vi "InitializeSystemHealthTags.vi"(8 "error in (no error)":errorcluster) -> (0 "error out":errorcluster, 3 "health tags":T1[](array[typedef]))   [LabVIEW 2017, in "DeviceHealth.lvlib"]
uses:
  <vilib>/addons/InsightCM/Devices/Shared/Common/DeviceHealth/DeviceHealth.lvlib
  <vilib>/addons/InsightCM/Devices/Shared/Common/DeviceHealth/controls/deviceHealthTag.ctl
  <vilib>/addons/InsightCM/Devices/Shared/Common/DeviceHealth/controls/SystemHealthTagEnum.ctl
  <vilib>/addons/InsightCM/MessageBus/Base/controls/Tag.ctl
  <vilib>/addons/InsightCM/MessageBus/Base/controls/KeyValuePair.ctl
  <vilib>/addons/InsightCM/Utilities/GlobalConfiguration/GlobalConfiguration.lvlib
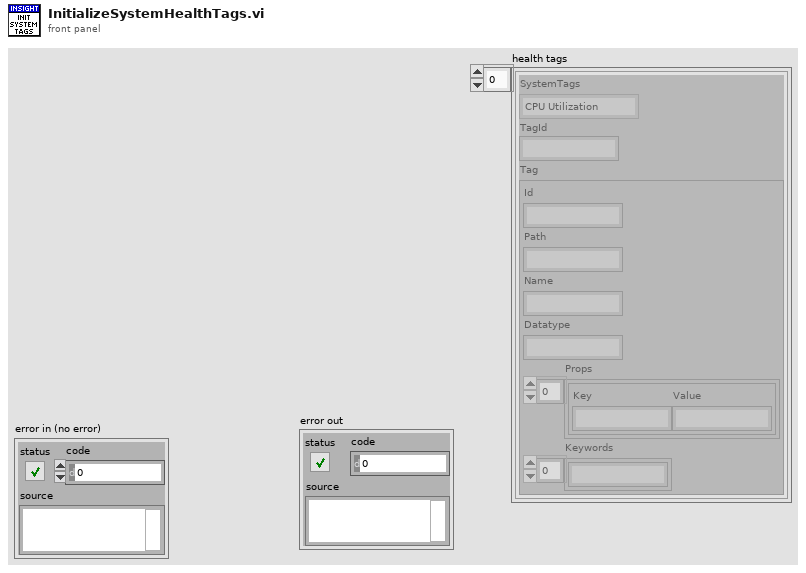
[diagram p1: front panel]
types:
  T1 = typedef "DeviceHealth.lvlib/deviceHealthTag.ctl" = cluster{"SystemTags":T2, "TagId":string, "Tag":T3}
  T2 = typedef "DeviceHealth.lvlib/SystemHealthTagEnum.ctl" = enum16{"CPU Utilization", "Memory Utilization", "Disk Utilization", "Total Physical Memory", "Primary Disk Free", "Chassis Temperature", "LowRateCount"}
  T3 = typedef "Tag.ctl" = cluster{"Id":string, "Path":string, "Name":string, "Datatype":string, "Props":T4[], "Keywords":string[]}
  T4 = typedef "KeyValuePair.ctl" = cluster{"Key":string, "Value":string}
  T5 = typedef "R2_Device.ctl" = cluster{"Id":string, "Name":string, "DeviceType":string, "HardwareName":string, "IpAddress":string, "HardwareInfo":T4[], "ApplicationType":string, "ApplicationVersion":string, "EquipmentIds":string[], "ConfigurationVersion":string, "State":T6, "Properties":T4[], "DataGroups":T7[], "BurstModeTrigger":T11}
  T6 = typedef "DeviceState.ctl" = cluster{"Disabled":bool}
  T7 = typedef "R2_DataGroup.ctl" = cluster{"Name":string, "OperatingStates":T8[], "Properties":T4[], "EquipmentIds":string[], "AssetNodeId":string}
  T8 = typedef "OperatingState.ctl" = cluster{"Name":string, "Properties":T4[], "Triggers":T9[]}
  T9 = typedef "Trigger.ctl" = cluster{"Type":string, "Expression":string, "Conditions":T10[]}
  T10 = typedef "Condition.ctl" = cluster{"Source":string, "Type":string, "Operator":string, "CompareTo":string, "DwellSeconds":dbl}
  T11 = typedef "BurstModeTrigger.ctl" = cluster{"Trigger":T9, "SampleRate":string, "AcquisitionLength":string}
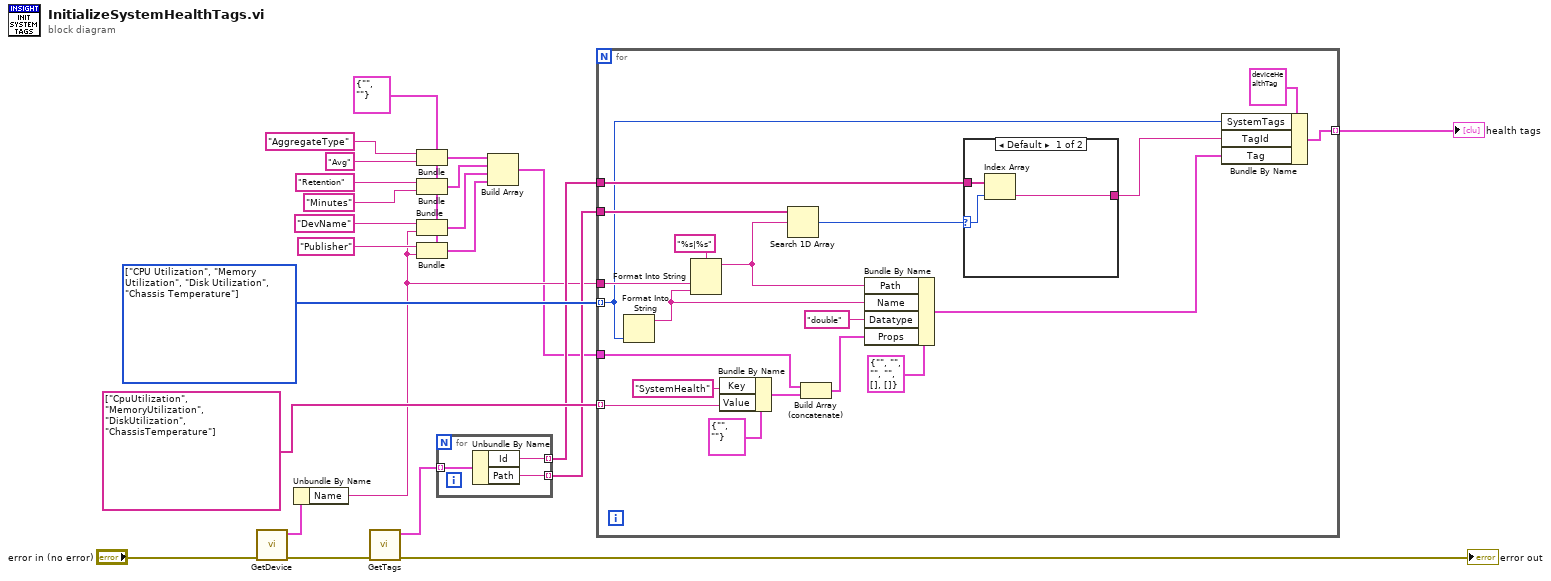
[diagram p0: block diagram]
diagram:
  w14 = T4 {"Key"="", "Value"=""}
  w23 = T2[] [enum."CPU Utilization", enum."Memory Utilization", enum."Disk Utilization", enum."Chassis Temperature"] items=["CPU Utilization", "Memory Utilization", "Disk Utilization", "Total Physical Memory", "Primary Disk Free", "Chassis Temperature", "LowRateCount"]
  n1 = call <vilib>:"GetDevice.vi"("error in (no error)"="error in (no error)") -> ("error out"=w19:errorcluster, "device configuration"=w21:T5)  [unwired: 8 in, 1 out]
  n2 = Unbundle By Name(w21) -> ("Name"=w3:string)
  n3 = call <vilib>:"GetTags.vi"("error in (no error)"=w19) -> ("error out"=→"error out":errorcluster, "tags"=w20:T3[])  [unwired: 8 in, 1 out]
  n4 = Bundle(cluster=w14, "Key"="AggregateType" ("SearchKey.Key"), "Value"="Avg" ("SearchKey.Key")) -> (w13:T4)
  n5 = Bundle(cluster=w14, "Key"="Retention" ("SearchKey.Key"), "Value"="Minutes" ("SearchKey.Key")) -> (w12:T4)
  n6 = Bundle(cluster=w14, "Key"="DevName" ("SearchKey.Key"), "Value"=w3) -> (w11:T4)
  n7 = Bundle(cluster=w14, "Key"="Publisher" ("SearchKey.Key"), "Value"=w3) -> (w10:T4)
  n8 = for {
    tunnel: w20 -> [w26] mode=indexing
    tunnel: [w25] -> w18 mode=indexing
    tunnel: [w24] -> w17 mode=indexing
    n9 = Unbundle By Name(w26) -> ("Id"=w24:string, "Path"=w25:string)
  }
  n10 = Build Array(w13, w12, w11, w10) -> (w2:T4[])
  n11 = for {
    tunnel: w23 -> [w31] mode=indexing
    tunnel: string[] ["CpuUtilization", "MemoryUtilization", "DiskUtilization", "ChassisTemperature"] -> [w43] mode=indexing
    tunnel: w3 -> [w40]
    tunnel: w18 -> [w36]
    tunnel: w17 -> [w33]
    tunnel: [w30] -> w16 mode=indexing
    tunnel: w2 -> [w29]
    n12 = Format Into String(w31) -> (resulting string=w38:string)  [unwired: 3 in, 1 out]
    n13 = Format Into String(format string="%s|%s", w40, w38) -> (resulting string=w35:string)  [unwired: 2 in, 1 out]
    n14 = Bundle By Name(cluster=T4 {"Key"="", "Value"=""}, "Key"="SystemHealth" ("SearchKey.Key"), "Value"=w43) -> (w42:T4)
    n15 = Search 1D Array(1D array=w36, element=w35) -> (index of element=w34:i32)  [unwired: 1 in]
    n16 = Build Array (concatenate)(w29, w42) -> (w41:T4[])
    n17 = Bundle By Name(cluster=T3 {"Id"="", "Path"="", "Name"="", "Datatype"="", "Props"=[], "Keywords"=[]} ("Tag"), "Path"=w35, "Name"=w38, "Datatype"="double", "Props"=w41) -> (w27:T3)
    n18 = case shown="Default" w34 {
      selector: w34 -> [w49 _]
      tunnel: w33 -> [w48 _]
      tunnel: [w47 _] -> w28
      frame Default {
        n19 = Index Array(array=w48, index=w49) -> (element=w47:string)
      }
      frame -1 {
      }
    }
    n20 = Bundle By Name(cluster=T1 {"SystemTags"=enum."CPU Utilization", "TagId"="", "Tag"={"Id"="", "Path"="", "Name"="", "Datatype"="", "Props"=[], "Keywords"=[]}} ("DeviceHealthTag"), "SystemTags"=w31, "TagId"=w28, "Tag"=w27) -> (w30:T1)
  }
  "health tags" <- w16
